vi "Add Actor Library to Project.vi"(7 "Application":refnum<vi>, 8 "error in (no error)":errorcluster, 9 "Library Path":path, 10 "Target Item":refnum<vi>) -> (0 "error out":errorcluster, 1 "Library out":refnum<vi>)   [LabVIEW 2023, in "Add Async Methods Actor.lvlib"]
uses:
  Add Async Methods Actor.lvlib
  Localized Strings.vi
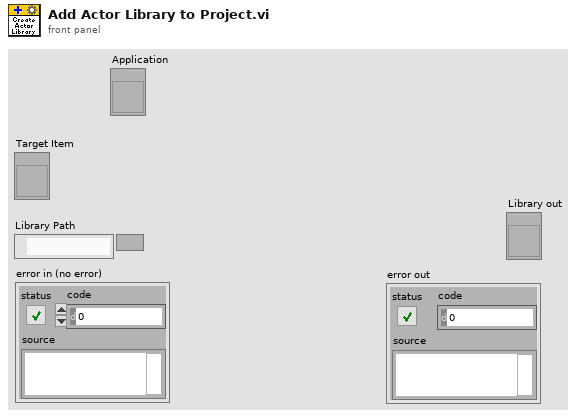
[diagram p1: front panel]
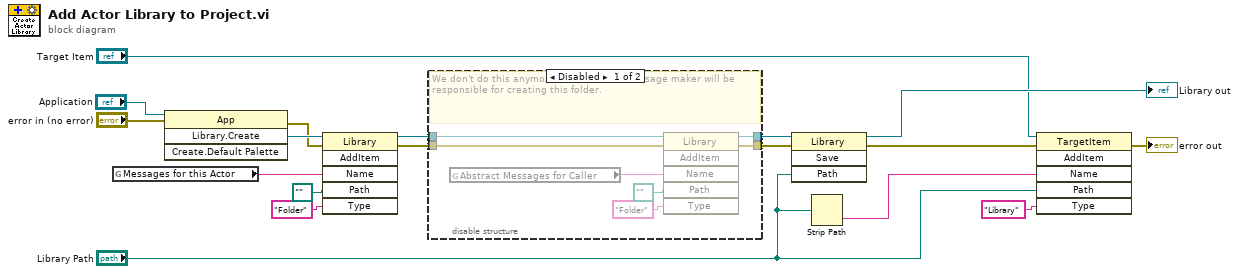
[diagram p0: block diagram]
diagram:
  n1 = global read "Localized Strings.vi" "Messages for this Actor"() -> (w4:string)
  n2 = invoke class="App" method="Library.Create"(reference="Application", error in="error in (no error)") -> (error out=w9:errorcluster, "Create Library"=w17:refnum<vi>)  [unwired: 2 in, 2 out]
  n3 = invoke class="Library" method="AddItem"(reference=w17, error in=w9, "Name"=w4, "Path"=path "", "Type"="Folder") -> (reference out=w6:refnum<vi>, error out=w7:errorcluster)  [unwired: 1 in, 4 out]
  n4 = disable-structure shown="Disabled" {
    disable-tunnel: [w23 w27] -> w8
    disable-tunnel: w7 -> [w22 w27]
    disable-tunnel: w6 -> [w21 w26]
    disable-tunnel: [w20 w26] -> w5
    frame Disabled {
      # "We don't do this anymore. The abstract message maker will be responsible for creating this folder."
      n5 = global read "Localized Strings.vi" "Abstract Messages for Caller"() -> (w19:string)
      n6 = invoke class="Library" method="AddItem"(reference=w21, error in=w22, "Name"=w19, "Path"=path "", "Type"="Folder") -> (reference out=w20:refnum<vi>, error out=w23:errorcluster)  [unwired: 1 in, 4 out]
    }
    frame Enabled {
    }
  }
  n7 = invoke class="Library" method="Save"(reference=w5, error in=w8, "Path"="Library Path") -> (reference out=→"Library out":refnum<vi>, error out=w12:errorcluster)  [unwired: 1 in, 2 out]
  n8 = Strip Path(path="Library Path") -> (name=w10:string)  [unwired: 1 out]
  n9 = invoke class="TargetItem" method="AddItem"(reference="Target Item", error in=w12, "Name"=w10, "Path"="Library Path", "Type"="Library") -> (error out=→"error out":errorcluster)  [unwired: 1 in, 5 out]
